vi "Stats2Strings.vi"(2 "stats":dbl[](array[numeric])) -> (7 "Strings":string[](array[string]))   [LabVIEW 2014]
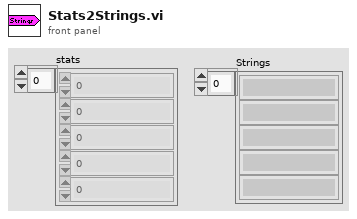
[diagram p1: front panel]
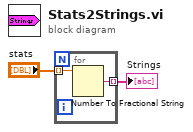
[diagram p0: block diagram]
diagram:
  n1 = for {
    tunnel: [w4] -> w1 mode=indexing
    tunnel: "stats" -> [w3] mode=indexing
    n2 = Number To Fractional String(number=w3) -> (F-format string=w4:string)  [unwired: 3 in]
  }
  "Strings" <- w1
